vi "Demo_Read_2.vi"() -> ()   [LabVIEW 2018]
panel:
  out "delimiter (Tab)":string
  out "reversed array":string[](array[string])
  out "array":string[](array[string])
  out "prompt (Open existing file)":string
  out "appended path":path
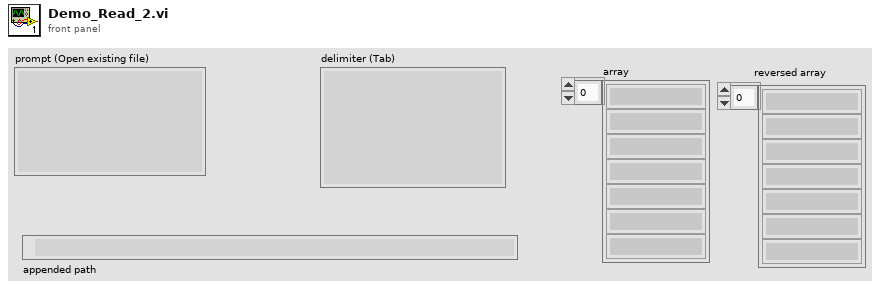
[diagram p1: front panel]
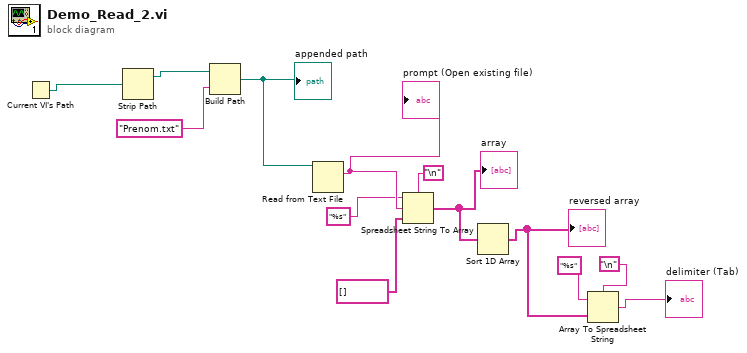
[diagram p0: block diagram]
diagram:
  n1 = Current VI's Path() -> (path=w13:path)
  n2 = Strip Path(path=w13) -> (stripped path=w1:path)  [unwired: 1 out]
  n3 = Build Path(base path=w1, name or relative path="Prenom.txt") -> (appended path=w11:path)
  "appended path" <- w11
  n4 = Read from Text File(file (use dialog)=w11) -> (text=w10:string)  [unwired: 3 in, 3 out]
  "prompt (Open existing file)" <- w10
  n5 = Spreadsheet String To Array(delimiter (Tab)="\n", format string="%s" ("spreadsheet string"), spreadsheet string=w10, array type (2D Dbl)=string[] [] ("spreadsheet string")) -> (array=w6:string[])
  "array" <- w6
  n6 = Sort 1D Array(array=w6) -> (sorted array=w5:string[])
  "reversed array" <- w5
  n7 = Array To Spreadsheet String(delimiter (Tab)="\n", array=w5, 3:"%s" ("delimiter (Tab)")) -> (spreadsheet string=→"delimiter (Tab)":string)
